vi "Disconnect.vi"(8 "error in (no error)":errorcluster, 11 "reference in":refnum<class "CR slave.lvclass">) -> (0 "error out":errorcluster, 3 "reference out":refnum<class "CR slave.lvclass">)   [LabVIEW 2019, in "CommandResponse communication.lvlib" / "CR slave.lvclass"]
doc: "Close all network streams to slave"
uses:
  CR slave.lvclass
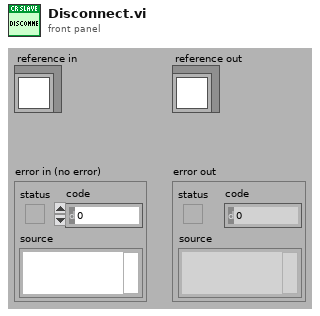
[diagram p1: front panel]
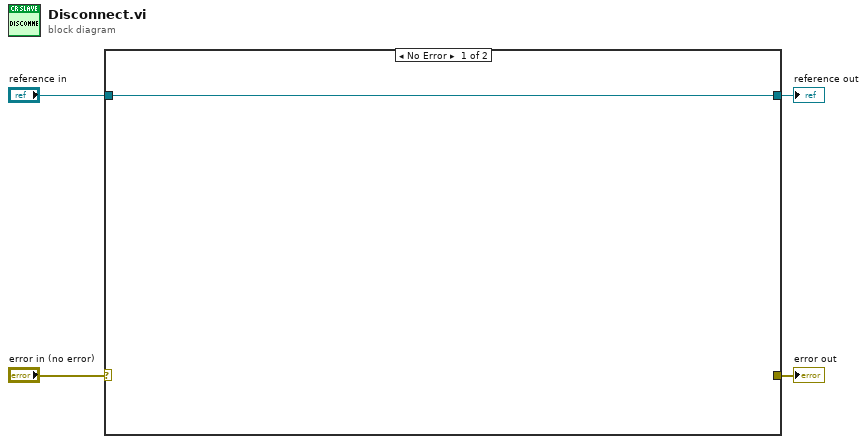
[diagram p0: block diagram]
diagram:
  n1 = case shown="No Error" "error in (no error)" {
    selector: "error in (no error)" -> [_ w7]
    tunnel: [_ w7] -> w3
    tunnel: [w5 w6] -> w1
    tunnel: "reference in" -> [w5 w6]
    frame No Error {
    }
    frame Error {
    }
  }
  "error out" <- w3
  "reference out" <- w1
